vi "CustomizeSetting.vi"(6 "タブ制御器ref":refnum<vi>, 8 "err(in)":errorcluster) -> (0 "err(out)":errorcluster)   [LabVIEW 2014]
uses:
  <vilib>/Utility/file.llb/Write To Spreadsheet File (string).vi
  <vilib>/Utility/file.llb/Read From Spreadsheet File (string).vi
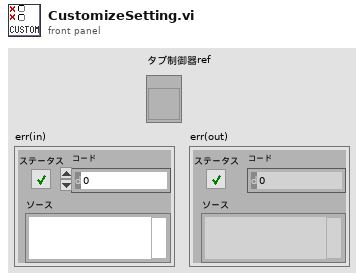
[diagram p1: front panel]
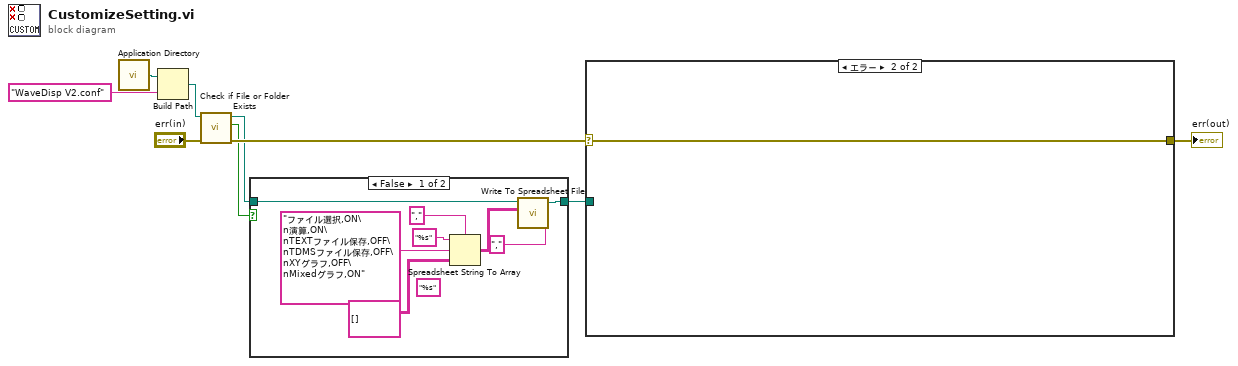
[diagram p0: block diagram]
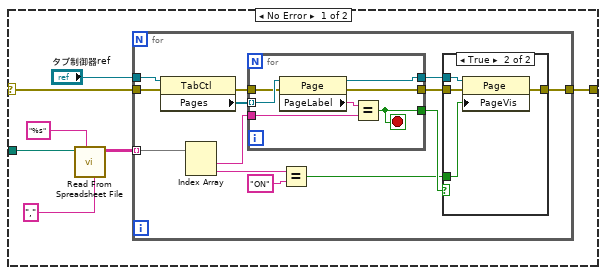
[diagram p3: hidden frame]
diagram:
  n1 = call <vilib>:"Application Directory.vi"() -> ("Application Directory"=w9:path)
  n2 = Build Path(base path=w9, name or relative path="WaveDisp V2.conf" ("名前または相対パス")) -> (appended path=w5:path)
  n3 = call <vilib>:"Check if File or Folder Exists.vi"("error in (no error)"="err(in)", "path"=w5) -> ("error out"=w4:errorcluster, "file or folder exists?"=w3:bool, "dup path"=w2:path)  [unwired: 7 in]
  n4 = case shown="FALSE" w3 {
    tunnel: w2 -> [w11 w18]
    tunnel: [w10 w18] -> w1
    frame False {
      (unwired) "%s" ("format (%s)")
      n5 = Spreadsheet String To Array(delimiter (Tab)="," ("デリミタ（タブ）"), format string="%s" ("形式文字列"), spreadsheet string="ファイル選択,ON\n演算,ON\nTEXTファイル保存,OFF\nTDMSファイル保存,OFF\nXYグラフ,OFF\nMixedグラフ,ON", array type (2D Dbl)=string[][] []) -> (array=w12:string[][])
      n6 = call-poly <vilib>:"Write To Spreadsheet File.vi"("delimiter (\\t)"="," ("delimiter (\\t)"), "2D data"=w12, "file path (dialog if empty)"=w11) -> ("new file path (Not A Path if cancelled)"=w10:path)  [unwired: 5 in]
    }
    frame True {
    }
  }
  n7 = case shown="エラー" w4 {
    selector: w4 -> [w19 w51]
    tunnel: [w22 w51] -> w8
    tunnel: w1 -> [w21 _]
    frame No Error {
      n8 = call-poly <vilib>:"Read From Spreadsheet File.vi"("delimiter (\\t)"="," ("delimiter (\\t)"), "format (%s)"="%s", "file path (dialog if empty)"=w21) -> ("all rows"=w25:string[][])  [unwired: 4 in, 4 out]
      n9 = for {
        tunnel: w25 -> [w38] mode=indexing
        tunnel: "タブ制御器ref" -> [w37]
        tunnel: w19 -> [w29]
        tunnel: [w26] -> w22
        n10 = property class="TabCtl"(reference=w37, error in=w29) -> (error out=w28:errorcluster, "Pages"=w36:refnum<vi>[])  [unwired: 1 out]
        n11 = Index Array(array=w38) -> (element #1=w35:string, element #2=w31:string)  [unwired: 2 in]
        n12 = for {
          tunnel: w36 -> [w50] mode=indexing
          tunnel: w35 -> [w48]
          tunnel: [w47] -> w33
          tunnel: [w46] -> w34
          tunnel: w28 -> [w45]
          tunnel: [w44] -> w27
          stop <- w46 stop-if-true
          n13 = property class="Page"(reference=w50, error in=w45) -> (reference out=w47:refnum<vi>, error out=w44:errorcluster, "PageLabel"=w49:string)
          n14 = Equal?(x=w49, y=w48) -> (x = y?=w46:bool)
        }
        n15 = Equal?(x=w31, y="ON") -> (x = y?=w30:bool)
        n16 = case shown="TRUE" w34 {
          tunnel: w33 -> [_ w43]
          tunnel: w30 -> [_ w42]
          tunnel: w27 -> [w39 w41]
          tunnel: [w39 w40] -> w26
          frame False {
          }
          frame True {
            n17 = property class="Page"(reference=w43, error in=w41, "PageVis"=w42) -> (error out=w40:errorcluster)  [unwired: 1 out]
          }
        }
      }
    }
    frame Error {
    }
  }
  "err(out)" <- w8
